vi "Read Instantiated by ref_.vi"(8 "error in (no error)":errorcluster, 11 "LV RT in":refnum<class "LV RT.lvclass">) -> (0 "error out":errorcluster, 2 "Instantiated by ref?":bool, 3 "LV RT out":refnum<class "LV RT.lvclass">)   [LabVIEW 2019, in "LV RT.lvclass"]
uses:
  LV RT.lvclass
  LV RT.lvclass/LV RT.ctl
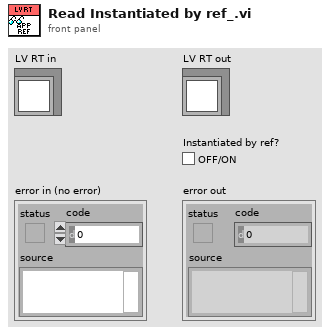
[diagram p1: front panel]
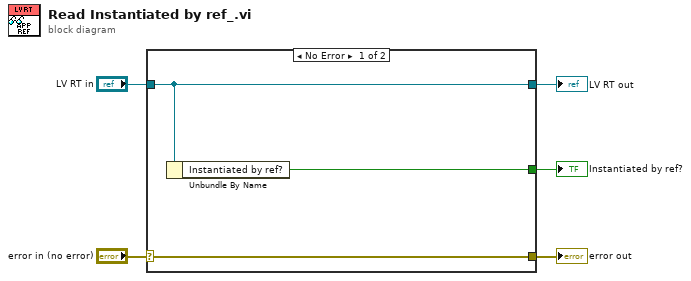
[diagram p0: block diagram]
diagram:
  n1 = case shown="No Error" "error in (no error)" {
    selector: "error in (no error)" -> [w8 w9]
    tunnel: [w8 w9] -> w4
    tunnel: [w7 w10] -> w2
    tunnel: "LV RT in" -> [w7 w10]
    tunnel: [w6 _] -> w1
    frame No Error {
      n2 = Unbundle By Name(w7) -> ("Instantiated by ref?"=w6:bool)
    }
    frame Error {
    }
  }
  "error out" <- w4
  "LV RT out" <- w2
  "Instantiated by ref?" <- w1
